vi "Calculate Test Coverage.vi"(6 "Ignore user.lib":bool, 8 "Ignore vi.lib":bool, 9 "Ignore non VIs":bool, 10 "Test Members":path[](array[path]), 11 "Project Members":path[](array[path])) -> (0 "% Coverage":dbl, 1 "Unused VI Count":i32, 2 "VI Names without coverage":string[](array[string]), 3 "VIs without coverage":path[](array[path]), 4 "Test VI Count":i32)   [LabVIEW 2009, in "GraphicalTestRunner.lvlib"]
uses:
  GraphicalTestRunner.lvlib
  <userlib>/_OpenG.lib/array/array.llb/Reorder 1D Array2 (Path)__ogtk.vi
  <userlib>/_OpenG.lib/array/array.llb/Sort 1D Array (String)__ogtk.vi
  <userlib>/_OpenG.lib/array/array.llb/Conditional Auto-Indexing Tunnel (Path)__ogtk.vi
  <userlib>/_OpenG.lib/file/file.llb/Strip Path Extension - Path__ogtk.vi
panel:
  # "Copyright © 2007 James Kring, Inc. All rights reserved.\n\nAuthor: Omar Mussa [omar.mussa@jameskring.com]\n\nThis library is provided \"AS IS\" ,WITHOUT WARRANTIES OR \nCONDITIONS OF ANY KIND, either express or implied.\n\nJames Kring, Inc. -- http://www.jameskring.com"
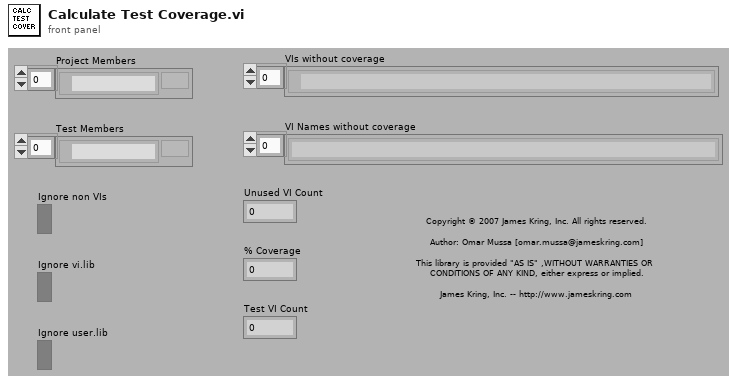
[diagram p1: front panel]
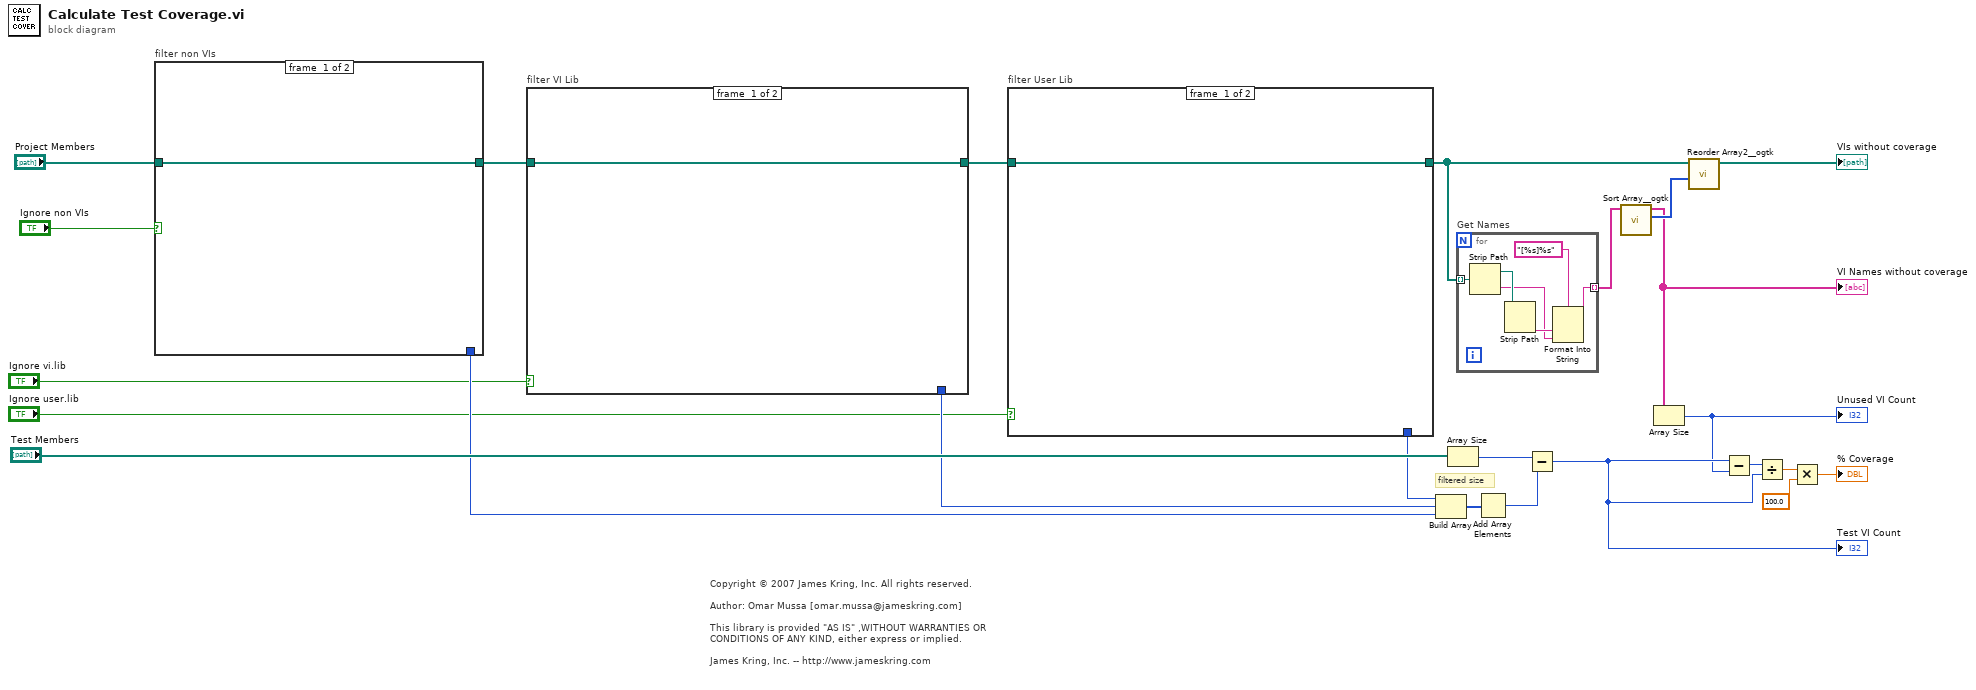
[diagram p0: block diagram]
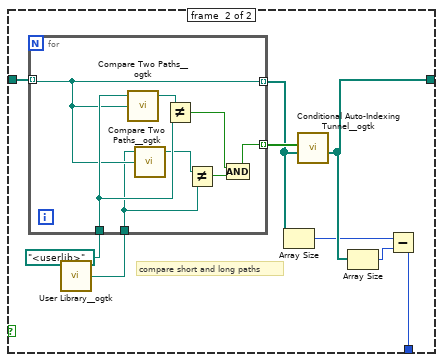
[diagram p2: hidden frame]
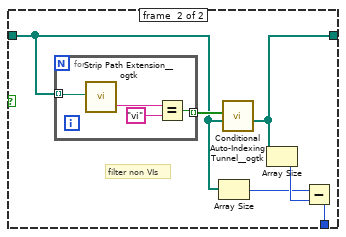
[diagram p3: hidden frame]
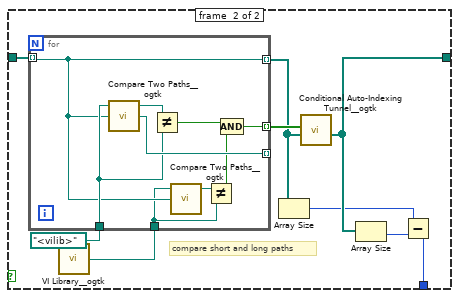
[diagram p4: hidden frame]
diagram:
  # "Copyright © 2007 James Kring, Inc. All rights reserved.\n\nAuthor: Omar Mussa [omar.mussa@jameskring.com]\n\nThis library is provided \"AS IS\" ,WITHOUT WARRANTIES OR \nCONDITIONS OF ANY KIND, either express or implied.\n\nJames Kring, Inc. -- http://www.jameskring.com"
  # "filtered size"
  n1 = case "filter non VIs" shown="True" "Ignore non VIs" {
    tunnel: "Project Members" -> [w25 w29]
    tunnel: [w25 w30] -> w4
    tunnel: [_ w26] -> w14
    frame #0 {
    }
    frame #1 {
      # "filter non VIs"
      n2 = for {
        tunnel: w29 -> [w35] mode=indexing
        tunnel: [w32] -> w31 mode=indexing
        n3 = call-poly <userlib>:"Strip Path Extension__ogtk.vi"("path"=w35) -> ("extension"=w34:string)  [unwired: 1 out]
        n4 = Equal?(x=w34, y="vi") -> (x = y?=w32:bool)
      }
      n5 = Array Size(array=w29) -> (size(s)=w27:i32)
      n6 = call-poly <userlib>:"Conditional Auto-Indexing Tunnel__ogtk.vi"("Array in"=w29, "Elements to keep"=w31) -> ("Filtered Array out"=w30:path[])  [unwired: 5 in]
      n7 = Array Size(array=w30) -> (size(s)=w28:i32)
      n8 = Subtract(x=w27, y=w28) -> (x-y=w26:i32)
    }
  }
  n9 = case "filter VI Lib" shown="True" "Ignore vi.lib" {
    tunnel: w4 -> [w36 w45]
    tunnel: [w36 w43] -> w5
    tunnel: [_ w40] -> w13
    frame #0 {
    }
    frame #1 {
      # "compare short and long paths"
      n10 = call <userlib>:"VI Library__ogtk.vi"() -> ("VI Library (+ Relative)"=w37:path)  [unwired: 1 in]
      n11 = for {
        tunnel: w45 -> [w51] mode=indexing
        tunnel: [w46] -> w44 mode=indexing
        tunnel: [w51] -> w39 mode=indexing
        tunnel: [w53] -> _ mode=indexing
        tunnel: path "<vilib>" ("VI Library (+ Relative)") -> [w52]
        tunnel: w37 -> [w49]
        n12 = call <userlib>:"Compare Two Paths__ogtk.vi"("path2"=w51, "path1"=w52) -> ("relative path from 1 to 2"=w53:path, "common path"=w54:path)  [unwired: 1 in, 1 out]
        n13 = Not Equal?(x=w54, y=w52) -> (x != y?=w47:bool)
        n14 = call <userlib>:"Compare Two Paths__ogtk.vi"("path2"=w51, "path1"=w49) -> ("common path"=w50:path)  [unwired: 1 in, 2 out]
        n15 = Not Equal?(x=w50, y=w49) -> (x != y?=w48:bool)
        n16 = Compound Arithmetic op=AND(w47, w48) -> (w46:bool)
      }
      n17 = Array Size(array=w39) -> (size(s)=w41:i32)
      n18 = call-poly <userlib>:"Conditional Auto-Indexing Tunnel__ogtk.vi"("Array in"=w39, "Elements to keep"=w44) -> ("Filtered Array out"=w43:path[])  [unwired: 5 in]
      n19 = Array Size(array=w43) -> (size(s)=w42:i32)
      n20 = Subtract(x=w41, y=w42) -> (x-y=w40:i32)
    }
  }
  n21 = case "filter User Lib" shown="True" "Ignore user.lib" {
    tunnel: w5 -> [w55 w64]
    tunnel: [w55 w62] -> w24
    tunnel: [_ w59] -> w12
    frame #0 {
    }
    frame #1 {
      # "compare short and long paths"
      n22 = call <userlib>:"User Library__ogtk.vi"() -> ("User Library (+ Relative)"=w56:path)  [unwired: 1 in]
      n23 = for {
        tunnel: w64 -> [w70] mode=indexing
        tunnel: [w65] -> w63 mode=indexing
        tunnel: [w70] -> w58 mode=indexing
        tunnel: path "<userlib>" ("VI Library (+ Relative)") -> [w71]
        tunnel: w56 -> [w68]
        n24 = call <userlib>:"Compare Two Paths__ogtk.vi"("path2"=w70, "path1"=w71) -> ("common path"=w72:path)  [unwired: 1 in, 2 out]
        n25 = call <userlib>:"Compare Two Paths__ogtk.vi"("path2"=w70, "path1"=w68) -> ("common path"=w69:path)  [unwired: 1 in, 2 out]
        n26 = Not Equal?(x=w72, y=w71) -> (x != y?=w66:bool)
        n27 = Not Equal?(x=w69, y=w68) -> (x != y?=w67:bool)
        n28 = Compound Arithmetic op=AND(w66, w67) -> (w65:bool)
      }
      n29 = Array Size(array=w58) -> (size(s)=w60:i32)
      n30 = call-poly <userlib>:"Conditional Auto-Indexing Tunnel__ogtk.vi"("Array in"=w58, "Elements to keep"=w63) -> ("Filtered Array out"=w62:path[])  [unwired: 5 in]
      n31 = Array Size(array=w62) -> (size(s)=w61:i32)
      n32 = Subtract(x=w60, y=w61) -> (x-y=w59:i32)
    }
  }
  n33 = Build Array(w12, w13, w14) -> (w15:i32[])
  n34 = Array Size(array="Test Members") -> (size(s)=w17:i32)
  n35 = for "Get Names" {
    tunnel: w24 -> [w78] mode=indexing
    tunnel: [w74] -> w20 mode=indexing
    n36 = Strip Path(path=w78) -> (stripped path=w77:path, name=w75:string)
    n37 = Strip Path(path=w77) -> (name=w76:string)  [unwired: 1 out]
    n38 = Format Into String(format string="[%s]%s", w76, w75) -> (resulting string=w74:string)  [unwired: 2 in, 1 out]
  }
  n39 = Add Array Elements(numeric array=w15) -> (sum=w16:i32)
  n40 = Subtract(x=w17, y=w16) -> (x-y=w18:i32)
  "Test VI Count" <- w18
  n41 = call-poly <userlib>:"Sort Array__ogtk.vi"("Array in"=w20) -> ("Sorted Pointers"=w22:i32[], "Sorted Array out"=w21:string[])  [unwired: 9 in]
  "VI Names without coverage" <- w21
  n42 = Array Size(array=w21) -> (size(s)=w7:i32)
  "Unused VI Count" <- w7
  n43 = call-poly <userlib>:"Reorder Array2__ogtk.vi"("indices"=w22, "array"=w24) -> ("reordered array"=→"VIs without coverage":path[])  [unwired: 9 in]
  n44 = Subtract(x=w18, y=w7) -> (x-y=w8:i32)
  n45 = Divide(x=w8, y=w18) -> (x/y=w9:dbl)
  n46 = Multiply(x=w9, y=100.0) -> (x*y=→"% Coverage":dbl)
